vi "Temperature Sensing.vi"() -> ()   [LabVIEW 2020]
panel:
  out "Blank Button 3":bool caption="fgjfj"
  in  "stop":bool
  out "Blank Button 2":bool caption="fgjfj"
  out "Blank Button":bool caption="fgjfj"
  out "Low Temp":bool
  out "Moderate Temp":bool
  out "High temp":bool
  out "Gauge":dbl(knob) caption="Temp" scale=-20.0..50.0
  out "Temp":dbl
  in  "Temperature Sensor":dbl(slide) scale=-20.0..50.0
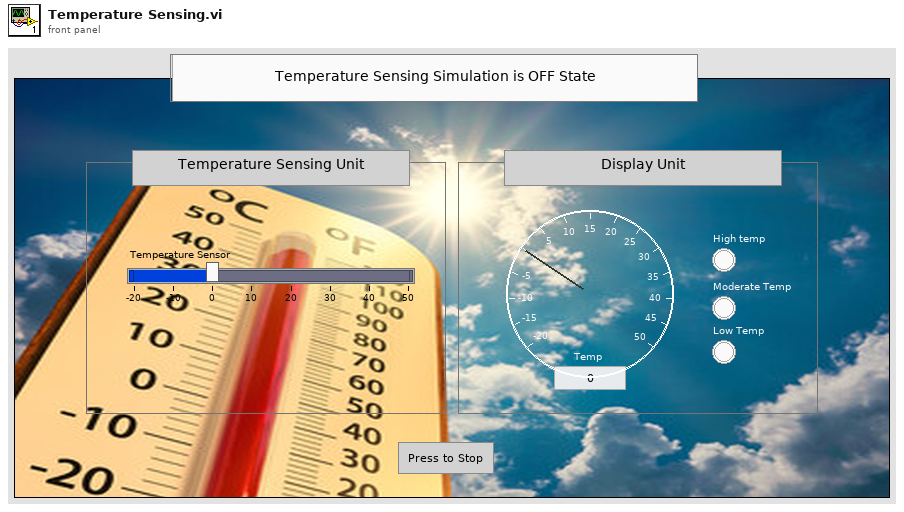
[diagram p1: front panel]
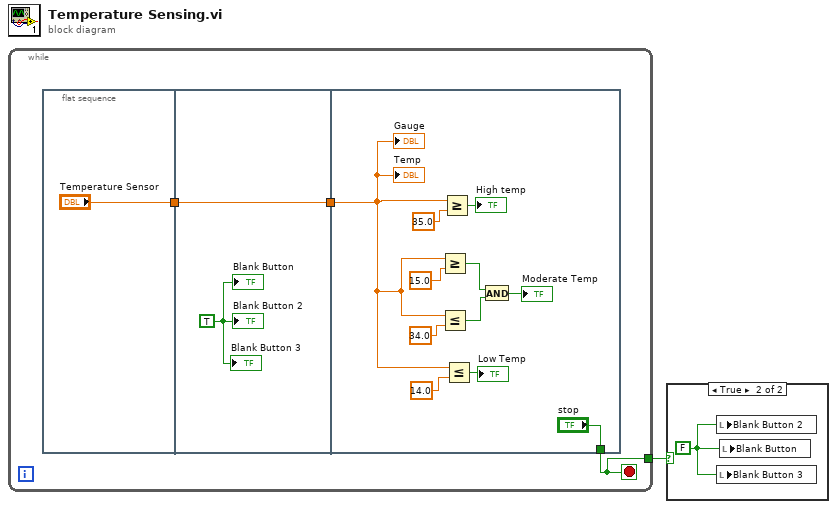
[diagram p0: block diagram]
diagram:
  n1 = while {
    tunnel: [w2] -> w1
    stop <- w2 stop-if-true
    n2 = flat-sequence {
      tunnel: ["Temperature Sensor"] -> w4
      tunnel: w4 -> [w7]
      tunnel: [w7] -> w3
      tunnel: w3 -> [w9]
      tunnel: ["stop"] -> w2
      frame #0 {
      }
      frame #1 {
        w6 = TRUE
        "Blank Button" <- w6
        "Blank Button 2" <- w6
        "Blank Button 3" <- w6
      }
      frame #2 {
        n3 = Greater Or Equal?(x=w9, y=15.0) -> (x >= y?=w15:bool)
        n4 = Less Or Equal?(x=w9, y=34.0) -> (x <= y?=w14:bool)
        n5 = Greater Or Equal?(x=w9, y=35.0) -> (x >= y?=→"High temp":bool)
        n6 = Less Or Equal?(x=w9, y=14.0) -> (x <= y?=→"Low Temp":bool)
        n7 = And(x=w15, y=w14) -> (x .and. y?=→"Moderate Temp":bool)
        "Temp" <- w9
        "Gauge" <- w9
      }
    }
  }
  n8 = case shown="True" w1 {
    frame False {
    }
    frame True {
      w19 = FALSE
      n9 = local write "Blank Button 2"(w19) -> ()
      n10 = local write "Blank Button 3"(w19) -> ()
      n11 = local write "Blank Button"(w19) -> ()
    }
  }
